vi "Example Serial 1.vi"() -> ()   [LabVIEW 2014]
uses:
  <vilib>/Aledyne-TSXperts/Arduino Compatible Compiler for LabVIEW/addons/Arduino SoftwareSerial Wrapper/Arduino SoftwareSerial Wrapper.lvlib
panel:
  out "Error Out":errorcluster
  in  "Error In":errorcluster
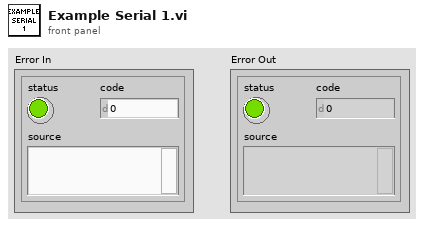
[diagram p1: front panel]
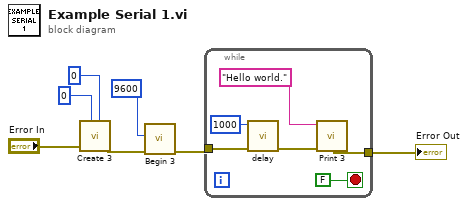
[diagram p0: block diagram]
diagram:
  n1 = call <vilib>:"Create 3.vi"("arduino RX pin"=u8 0, "arduino TX pin"=u8 0, "Error In"="Error In") -> ("Error Out"=w2:errorcluster)  [unwired: 8 in]
  n2 = call <vilib>:"Begin 3.vi"("Error In"=w2, "Baudrate"=u16 9600) -> ("Error Out"=w3:errorcluster)  [unwired: 8 in]
  n3 = while {
    tunnel: w3 -> [w12]
    tunnel: [w13] -> w6
    stop <- FALSE stop-if-true
    n4 = call "delay.vi"("Error In"=w12, "time (ms)"=1000) -> ("Error Out"=w11:errorcluster)  [unwired: 9 in]
    n5 = call <vilib>:"Print 3.vi"("Error In"=w11, "String to print"="Hello world.") -> ("Error Out"=w13:errorcluster)  [unwired: 9 in]
  }
  "Error Out" <- w6
